vi "ESN_evaluateByMSE.vi"   [LabVIEW 2017]
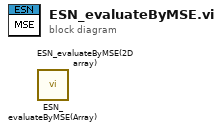
[diagram p0: block diagram]
diagram:
  n1 = call "ESN_evaluateByMSE(Array).vi"() -> ()  [unwired: 10 in, 2 out]
  n2 = call "ESN_evaluateByMSE(2D array).vi"() -> ()  [unwired: 10 in, 2 out]
